vi "clear Session Data.vi"(0 "OBJ - Measurement Session in":refnum<class "Data DVR Session.lvclass">, 11 "error in":errorcluster) -> (4 "OBJ - Measurement Session out":refnum<class "Data DVR Session.lvclass">, 15 "error out":errorcluster)   [LabVIEW 2015, in "Data DVR Session.lvclass"]
doc: "OVERRIDE VI\nPlaceholder for decendant classes to clear session information and close references."
uses:
  Data DVR Session.lvclass
  Data DVR Session.lvclass/Data DVR Session.ctl
  Data/Data.lvclass
  Read DVR.vi
  Write Data.vi
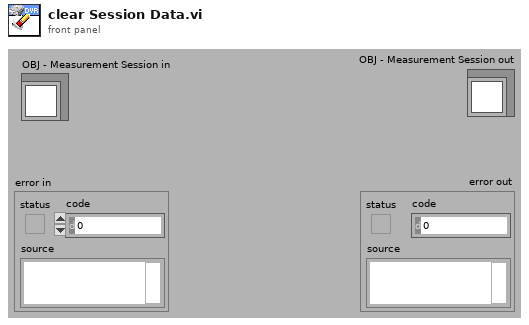
[diagram p1: front panel]
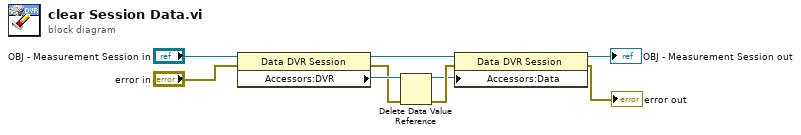
[diagram p0: block diagram]
diagram:
  n1 = property class="Data DVR Session"(reference="OBJ - Measurement Session in", error in="error in") -> (reference out=w4:refnum<class "Data DVR Session.lvclass">, error out=w6:errorcluster, "Accessors:DVR"=w8:refnum<data-value>)
  n2 = Delete Data Value Reference(data value reference=w8, error in=w6) -> (data value=w1:refnum<class "Data.lvclass">, error out=w3:errorcluster)
  n3 = property class="Data DVR Session"(reference=w4, error in=w3, "Accessors:Data"=w1) -> (reference out=→"OBJ - Measurement Session out":refnum<class "Data DVR Session.lvclass">, error out=→"error out":errorcluster)
